vi "IPC Flasher Main.vi"() -> ()   [LabVIEW 2021]
uses:
  <vilib>/xnet/xnet.llb/XNET Create Session (Signal Input Single-point).vi
panel:
  in  "New Message":string
  out "Console":string
  in  "Barcode":string="Barcode"
  in  "Run":bool
  in  "Stop":bool
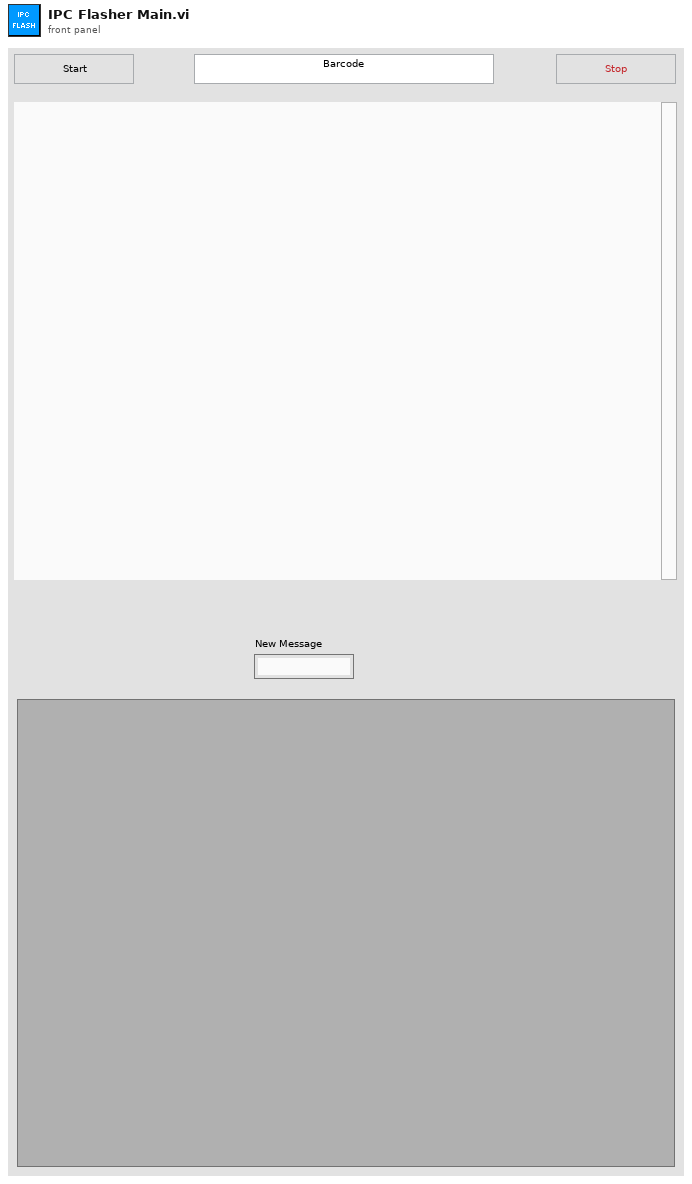
[diagram p1: front panel]
types:
  T1 = enum8{"Enabled", "Disabled", "Disabled and Grayed Out"}
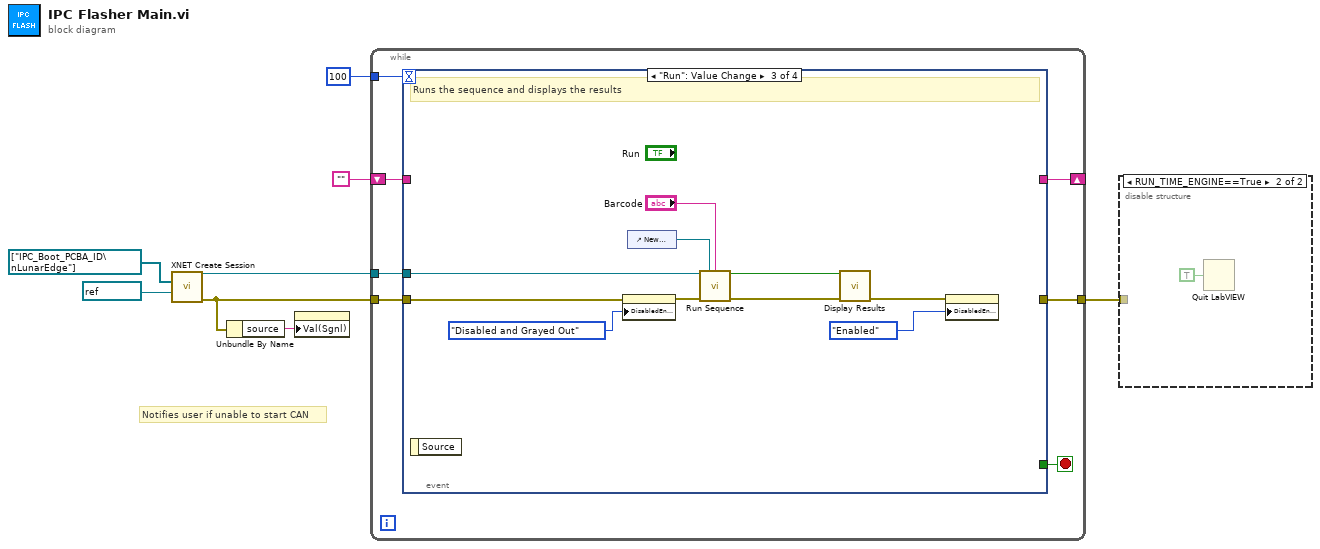
[diagram p0: block diagram]
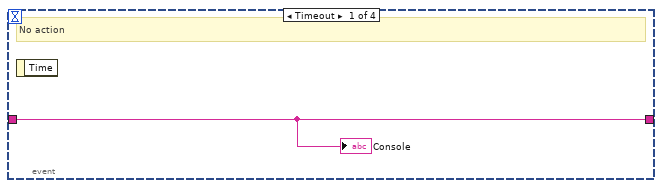
[diagram p3: hidden frame]
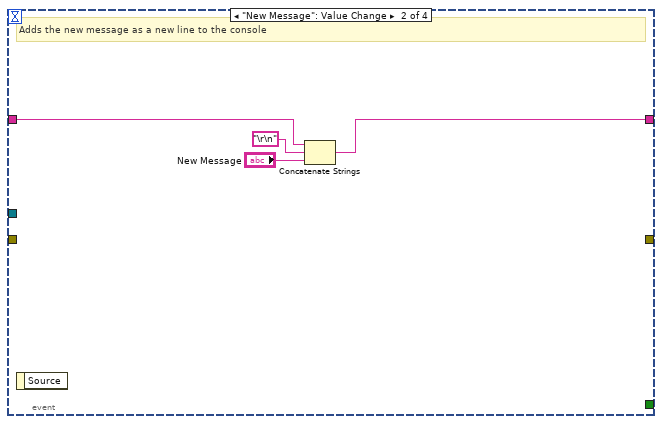
[diagram p4: hidden frame]
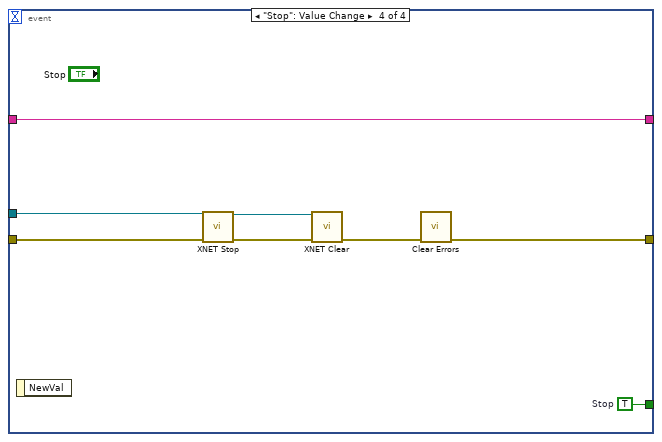
[diagram p5: hidden frame]
diagram:
  # "Notifies user if unable to start CAN"
  n1 = call-poly <vilib>:"XNET Create Session.vi"("signal list"=refnum<k21>[] ["IPC_Boot_PCBA_ID\nLunarEdge"], "interface"=refnum<k21> "CAN1") -> ("session out"=w4:refnum<k21>, "error out"=w3:errorcluster)  [unwired: 12 in]
  n2 = Unbundle By Name(w3) -> ("source"=w2:string)
  n3 = property on="New Message" class="Str"("Val(Sgnl)"=w2) -> ()  [unwired: 2 in, 2 out]
  n4 = while {
    tunnel: 100 -> [w15]
    shift-right: [w12] -> _
    shift-left: "" -> [w13]
    tunnel: w3 -> [w11]
    tunnel: w4 -> [w10]
    tunnel: [w9] -> w1
    stop <- w14 stop-if-true
    n5 = event shown="[2] \"Run\": Value Change" {
      selector: _ -> [_ _ _ _]
      dyn-events: _ -> [_ _ _ _]
      timeout: w15 -> [_ _ _ _]
      tunnel: [_ _ _ w38] -> w14
      tunnel: w13 -> [w16 w20 _ w37]
      tunnel: [w16 w17 _ w37] -> w12
      tunnel: w11 -> [_ _ w21 w36]
      tunnel: w10 -> [_ _ w28 w34]
      tunnel: [_ _ _ w31] -> w9
      event Timeout {
        # "No action"
        n6 = event-data() -> ()  [unwired: 1 in, 1 out]
        "Console" <- w16
      }
      event "New Message": Value Change {
        # "Adds the new message as a new line to the console"
        n7 = event-data() -> ()  [unwired: 1 in, 1 out]
        n8 = Concatenate Strings(w20, "\r\n", "New Message") -> (w17:string)
      }
      event "Run": Value Change {
        # "Runs the sequence and displays the results"
        n9 = event-data() -> ()  [unwired: 1 in, 1 out]
        n10 = property on="Run" class="Bool"(error in=w21, "DisabledEnum"=T1."Disabled and Grayed Out" ("Disabled")) -> (error out=w25:errorcluster)  [unwired: 1 in, 1 out]
        n11 = control-ref of="New Message"() -> (w27:refnum<vi>)
        n12 = call "Run Sequence.vi"("XNET Sesion"=w28, "Console"=w27, "Barcode"="Barcode", "Error In"=w25) -> ("Pass"=w30:bool, "Error Out"=w23:errorcluster)  [unwired: 10 in]
        n13 = call "Display Results.vi"("Error In"=w23, "Pass"=w30) -> ("Error Out"=w26:errorcluster)  [unwired: 9 in]
        n14 = property on="Run" class="Bool"(error in=w26, "DisabledEnum"=T1."Enabled" ("Disabled")) -> ()  [unwired: 1 in, 2 out]
      }
      event "Stop": Value Change {
        w38 = TRUE  # Stop
        n15 = event-data() -> ()  [unwired: 1 in, 1 out]
        n16 = call <vilib>:"XNET Stop.vi"("session in"=w34, "error in (no error)"=w36) -> ("session out"=w33:refnum<k21>, "error out"=w35:errorcluster)  [unwired: 12 in]
        n17 = call <vilib>:"XNET Clear.vi"("session in"=w33, "error in (no error)"=w35) -> ("error out"=w32:errorcluster)  [unwired: 13 in]
        n18 = call <vilib>:"Clear Errors.vi"("error in (no error)"=w32) -> ("error out"=w31:errorcluster)  [unwired: 5 in, 1 out]
      }
    }
  }
  n19 = disable-structure shown="RUN_TIME_ENGINE==True" {
    disable-tunnel: w1 -> [_ _]
    frame condition #0 (active) {
    }
    frame condition #1 {
      n20 = Quit LabVIEW(quit? (T)=TRUE) -> ()
    }
  }
